vi "Open File.vi"() -> (0 "error out":errorcluster, 3 "refnum out":refnum<file>)   [LabVIEW 2017]
doc: "Opens the .dat file with a reference number in the default My Documents\\LabVIEW Data directory.\n\nUse this VI is used as the setup VI for Read from File.lvtest."
panel:
  # "Overview: Use this VI as the setup VI for Write to File.lvtest.\nRequirements: LabVIEW Full Development System, Unit Test Framework Toolkit\nInstructions: \n1.  In the Project Explorer window, double-click Read from File.lvtest to display the Test Properties dialog box.\n2.  Select Setup/Teardown from the Category list to display the Setup/Teardown page. You can understand how LabVIEW passes the output value from the setup VI to the input of the VI under test."
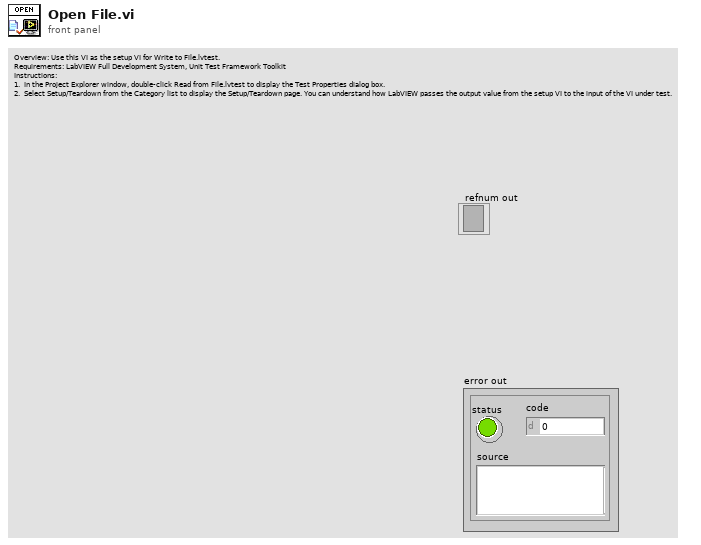
[diagram p1: front panel]
types:
  T1 = enum16{"open", "replace", "create", "open or create", "replace or create", "replace or create with confirmation"}
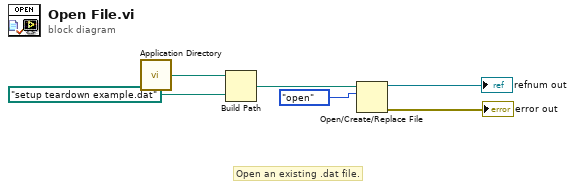
[diagram p0: block diagram]
diagram:
  # "Open an existing .dat file."
  n1 = call <vilib>:"Application Directory.vi"() -> ("Application Directory"=w3:path)
  n2 = Build Path(base path=w3, name or relative path=path "setup teardown example.dat") -> (appended path=w1:path)
  n3 = Open/Create/Replace File(file path (use dialog)=w1, operation (0:open)=T1."open") -> (refnum out=→"refnum out":refnum<file>, error out=→"error out":errorcluster)  [unwired: 1 in, 4 out]
